vi "Configure Modulation Low Level (FM Deviation).vi"(8 "error in":errorcluster, 10 "Peak Deviation (100.00 Hz)":dbl=100.0 min=1e-06 max=25050000.0, 11 "VISA resource name":refnum<visa-resource-name>) -> (0 "error out":errorcluster, 3 "VISA resource name out":refnum<visa-resource-name>)   [LabVIEW 2017, in "Keithley 3390.lvlib"]
doc: "Sets the frequency deviation for the frequency modulation technique. The frequency deviation represents the peak variation in the frequency of the modulation output based on that of the carrier wave."
uses:
  Keithley 3390.lvlib
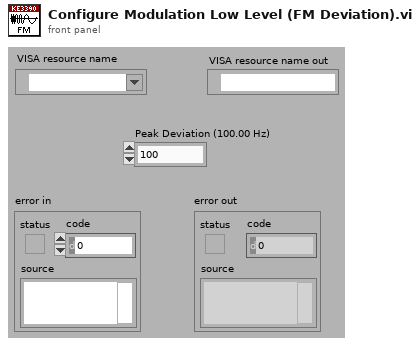
[diagram p1: front panel]
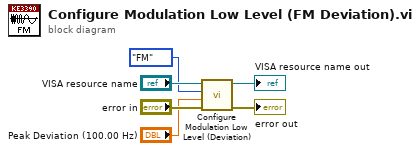
[diagram p0: block diagram]
diagram:
  n1 = call "Configure Modulation Low Level (Deviation).vi"("error in (no error)"="error in", "Deviation"="Peak Deviation (100.00 Hz)", "Modulation (FM)"=enum16{"FM", "PM", "PWM"}."FM" ("Modulation (0: FM)"), "VISA resource name"="VISA resource name") -> ("error out"=→"error out":errorcluster, "VISA resource name out"=→"VISA resource name out":refnum<visa-resource-name>)  [unwired: 6 in]
